vi "Finalize To Settings.vi"(8 "error in":errorcluster, 11 "RDMA Tx Transfer Configuration in":refnum<class "RDMA Transfer Tx Configuration.lvclass">=refnum) -> (0 "error out":errorcluster, 2 "settings":cluster{"key":string, "value":string}[](array[cluster]), 3 "RDMA Tx Transfer Configuration out":refnum<class "RDMA Transfer Tx Configuration.lvclass">)   [LabVIEW 2020, in "RDMA.lvlib" / "RDMA Transfer Tx Configuration.lvclass"]
uses:
  RDMA Transfer Tx Configuration.lvclass
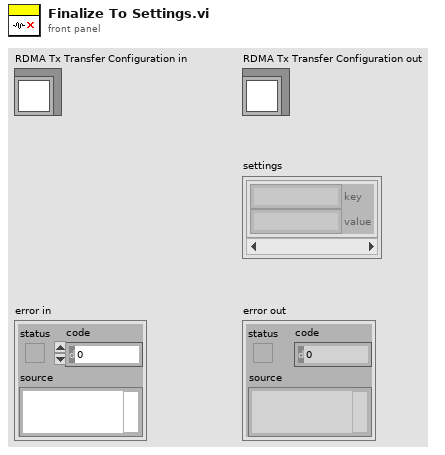
[diagram p1: front panel]
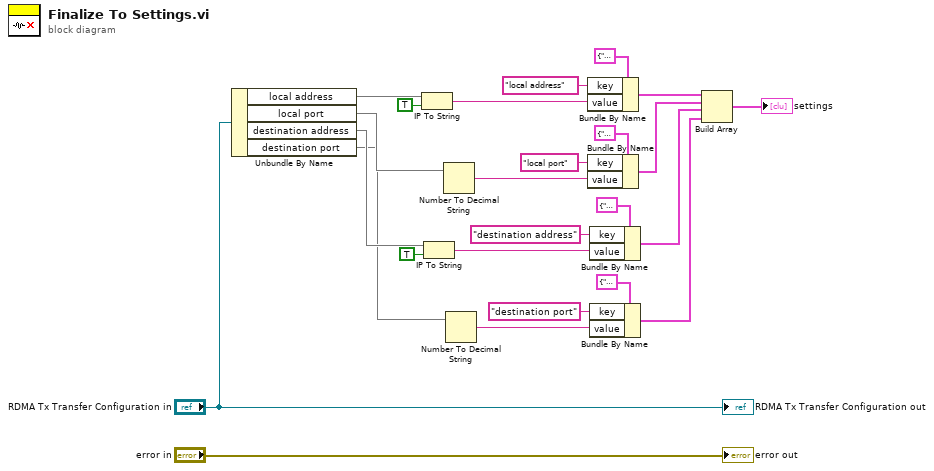
[diagram p0: block diagram]
diagram:
  n1 = Unbundle By Name("RDMA Tx Transfer Configuration in") -> ("local address"=w22, "local port"=w17, "destination address"=w8, "destination port"=w7)
  n2 = IP To String(1:TRUE ("dot notation? (F)"), 2:w22) -> (0:w20:string)
  n3 = IP To String(1:TRUE ("dot notation? (F)"), 2:w8) -> (0:w12:string)
  n4 = Number To Decimal String(number=w17) -> (decimal integer string=w16:string)  [unwired: 1 in]
  n5 = Number To Decimal String(number=w7) -> (decimal integer string=w15:string)  [unwired: 1 in]
  n6 = Bundle By Name(cluster=cluster{"key":string, "value":string} {"key"="", "value"=""} ("setting"), "key"="local address", "value"=w20) -> (w6:cluster{"key":string, "value":string})
  n7 = Bundle By Name(cluster=cluster{"key":string, "value":string} {"key"="", "value"=""} ("setting"), "key"="local port", "value"=w16) -> (w5:cluster{"key":string, "value":string})
  n8 = Bundle By Name(cluster=cluster{"key":string, "value":string} {"key"="", "value"=""} ("setting"), "key"="destination address", "value"=w12) -> (w4:cluster{"key":string, "value":string})
  n9 = Bundle By Name(cluster=cluster{"key":string, "value":string} {"key"="", "value"=""} ("setting"), "key"="destination port", "value"=w15) -> (w3:cluster{"key":string, "value":string})
  n10 = Build Array(w6, w5, w4, w3) -> (→"settings":cluster{"key":string, "value":string}[])
  "error out" <- "error in"
  "RDMA Tx Transfer Configuration out" <- "RDMA Tx Transfer Configuration in"
